vi "dc_motor_drive_pidff.vi"() -> ()   [LabVIEW 2019]
uses:
  <vilib>/myRIO/Common/Instrument Driver Framework/myRIO v1.0/Encoder/typedefs/Encoder Signal Mode.ctl
  <vilib>/myRIO/Instrument Drivers/Onboard IO/Encoder/typedefs/Encoder Reference.ctl
  <vilib>/myRIO/Common/Instrument Driver Framework/Utilities/typedefs/myRIO Generic Hardware Reference.ctl
  <vilib>/myRIO/Common/Instrument Driver Framework/Utilities/typedefs/Hardware Version Enum.ctl
  <vilib>/myRIO/Common/Instrument Driver Framework/Utilities/typedefs/myRIO v1.0 Reference.ctl
  <vilib>/myRIO/Common/Instrument Driver Framework/Utilities/typedefs/Generic FPGA Reference.ctl
  <vilib>/myRIO/Common/Instrument Driver Framework/myRIO v1.0/Encoder/typedefs/Encoder Channels Enum.ctl
  <vilib>/myRIO/Common/Instrument Driver Framework/myRIO v1.0/Encoder/typedefs/Encoder Configuration v1.0.ctl
  <vilib>/userDefined/High Color/nirio_resource_hc.ctl
  <vilib>/Platform/TimedLoop/XDataNode/timing_clust.ctl
  <vilib>/Platform/TimedLoop/XDataNode/nitl_modes.ctl
  <vilib>/Platform/TimedLoop/XDataNode/wakeup.ctl
  <vilib>/myRIO/Instrument Drivers/Onboard IO/PWM/typedefs/PWM Reference.ctl
  <vilib>/myRIO/Common/Instrument Driver Framework/myRIO v1.0/PWM/typedefs/PWM Channels Enum.ctl
  <vilib>/myRIO/Instrument Drivers/Onboard IO/PWM/typedefs/PWM Configuration.ctl
  <vilib>/myRIO/Instrument Drivers/Onboard IO/DIO/typedefs/DIO Reference.ctl
  <vilib>/myRIO/Common/Instrument Driver Framework/myRIO v1.0/DIO/typedefs/DIO Channels List.ctl
  <vilib>/myRIO/Common/Instrument Driver Framework/myRIO v1.0/DIO/typedefs/DIO Channels Enum.ctl
  <vilib>/myRIO/Common/Instrument Driver Framework/Utilities/vis/Is FPGA Ref Available.vi
  <vilib>/myRIO/Common/Instrument Driver Framework/myRIO v1.0/Encoder/vis/myRIO v1.1 Open Encoder.vi
  <vilib>/myRIO/Instrument Drivers/Onboard IO/Encoder/vis/Read.vi
  <vilib>/myRIO/Common/Instrument Driver Framework/myRIO v1.0/PWM/vis/myRIO v1.1 Open PWM.vi
  <vilib>/myRIO/Common/Instrument Driver Framework/myRIO v1.0/DIO/vis/myRIO v1.1 Open DIO.vi
  <vilib>/myRIO/Instrument Drivers/Onboard IO/DIO/vis/Write.vi
  <vilib>/myRIO/Common/Instrument Driver Framework/Utilities/vis/Validate Channels.vi
  <vilib>/myRIO/Common/Instrument Driver Framework/myRIO v1.0/Encoder/vis/myRIO v1.0 Reserve Encoder.vi
  <vilib>/myRIO/Common/Instrument Driver Framework/myRIO v1.0/PWM/vis/myRIO v1.0 Reserve PWM.vi
  <vilib>/myRIO/Common/Instrument Driver Framework/myRIO v1.0/DIO/vis/myRIO v1.0 Reserve DIO.vi
  <vilib>/myRIO/Common/Instrument Driver Framework/myRIO v1.0/Encoder/vis/myRIO v1.0 Build MUX Configuration Encoder.vi
  <vilib>/myRIO/Common/Instrument Driver Framework/myRIO v1.0/Resource Manager/vis/myRIO v1.0 Reserve Channel List.vi
  <vilib>/myRIO/Common/Instrument Driver Framework/myRIO v1.0/PWM/vis/myRIO v1.0 Build MUX Configuration PWM.vi
  <vilib>/myRIO/Common/Instrument Driver Framework/myRIO v1.0/DIO/vis/myRIO v1.0 Build MUX Configuration DIO.vi
  <vilib>/myRIO/Common/Instrument Driver Framework/myRIO v1.0/Resource Manager/vis/myRIO v1.0 Create Configuration List.vi
  <vilib>/myRIO/Common/Instrument Driver Framework/myRIO v1.0/Resource Manager/vis/myRIO v1.0 Reserve Channel.vi
  <vilib>/myRIO/Common/Instrument Driver Framework/myRIO v1.0/Resource Manager/vis/myRIO v1.0 Unreserve Channel.vi
  <vilib>/myRIO/Common/Instrument Driver Framework/myRIO v1.0/Resource Manager/vis/myRIO v1.0 Build Mutex Name.vi
  <vilib>/Utility/VariantDataType/GetNumericInfo.vi
  <vilib>/Utility/error.llb/Error Cluster From Error Code.vi
  <vilib>/myRIO/Common/Instrument Driver Framework/myRIO v1.0/myRIO v1.1 Open.vi
  <vilib>/myRIO/Common/Instrument Driver Framework/Utilities/vis/IO Manager.vi
  <vilib>/myRIO/Common/Instrument Driver Framework/Utilities/vis/Configuration Manager.vi
  <vilib>/myRIO/Common/Instrument Driver Framework/myRIO v1.0/Resource Manager/vis/myRIO v1.0 Configure IO.vi
  <vilib>/myRIO/Common/Instrument Driver Framework/myRIO v1.0/myRIO v1.0 Close.vi
  <vilib>/myRIO/Common/Instrument Driver Framework/myRIO v1.0/Encoder/vis/myRIO v1.0 Configure Encoder.vi
  <vilib>/myRIO/Common/Instrument Driver Framework/myRIO v1.0/Encoder/vis/myRIO v1.0 Read Encoder.vi
  <vilib>/myRIO/Common/Instrument Driver Framework/myRIO v1.0/PWM/vis/myRIO v1.0 Write PWM.vi
  <vilib>/myRIO/Common/Instrument Driver Framework/myRIO v1.0/DIO/vis/myRIO v1.0 Write DIO.vi
  <vilib>/myRIO/Express VI/Onboard IO/Encoder/Encoder Express VI.xnode
  <vilib>/myRIO/Instrument Drivers/Onboard IO/Encoder/vis/myRIO Encoder Open.xnode
  <vilib>/myRIO/Common/Instrument Driver Framework/myRIO v1.0/Encoder/typedefs/Encoder Count Direction Enum.ctl
  <vilib>/Platform/TimedLoop/XDataNode/XDataNode.xnode
  <vilib>/myRIO/Express VI/Onboard IO/PWM/PWM Express VI.xnode
  <vilib>/myRIO/Instrument Drivers/Onboard IO/PWM/vis/myRIO PWM Open.xnode
  <vilib>/myRIO/Express VI/Onboard IO/DO/DO Express VI.xnode
  <vilib>/myRIO/Instrument Drivers/Onboard IO/DIO/vis/myRIO DIO Open.xnode
  <vilib>/myRIO/Instrument Drivers/Onboard IO/PWM/PWM.lvlib
  <vilib>/myRIO/Instrument Drivers/Utilities/Utilities.lvlib
  <vilib>/myRIO/Instrument Drivers/Onboard IO/Encoder/Encoder.lvlib
  <vilib>/Platform/TimedLoop/XDataNode/XDNodeRunTimeDep.lvlib
  <vilib>/myRIO/Instrument Drivers/Onboard IO/DIO/DIO.lvlib
panel:
  out "direction":bool
  out "Angle diff(deg)":dbl(graph)
  out "virtual PWM value":dbl[](graph)
  out "Duty cycle":dbl(graph)
  out "PWM value":i32
  out "Set Point 2":dbl
  out "Set Point":dbl
  out "Setpoint_to_motor":T1
  in  "PWM Max":i32=4096
  in  "gain_ff":T2={"gain_ff 1"={"K_vff"=10000.0, "K_aff"=250.0}, "gain_ff 2"={"K_vff"=10000.0, "K_aff"=250.0}, "gain_ff 3"={"K_vff"=10000.0, "K_aff"=250.0}, "gain_ff 4"={"K_vff"=10000.0, "K_aff"=250.0}, "gain_ff 5"={"K_vff"=10000.0, "K_aff"=250.0}, "gain_ff 6"={"K_vff"=10000.0, "K_aff"=250.0}}
  in  "PIDt":T3={"PID gains 1"={"proportional gain (Kp)"=800.0, "integral time (Ki)"=0.0, "derivative time (Kd)"=1000.0}, "PID gains 2"={"proportional gain (Kp)"=800.0, "integral time (Ki)"=0.0, "derivative time (Kd)"=1000.0}, "PID gains 3"={"proportional gain (Kp)"=800.0, "integral time (Ki)"=0.0, "derivative time (Kd)"=1000.0}, "PID gains 4"={"proportional gain (Kp)"=800.0, "integral time (Ki)"=0.0, "derivative time (Kd)"=1000.0}, "PID gains 5"={"proportional gain (Kp)"=800.0, "integral time (Ki)"=0.0, "derivative time (Kd)"=1000.0}, "PID gains 6"={"proportional gain (Kp)"=800.0, "integral time (Ki)"=0.0, "derivative time (Kd)"=1000.0}}
  in  "PWM value":T4 {"PWM value 6" scale=0.0..4096.0; "PWM value 5" scale=0.0..4096.0; "PWM value 4" scale=0.0..4096.0; "PWM value 3" scale=0.0..4096.0; "PWM value 2" scale=0.0..4096.0; "PWM value 1" scale=0.0..4096.0}
  out "time":dbl
  out "Angle_velocity(deg/s)":cluster{"set point":dbl, dbl}(graph)
  out "Angle_velocity(deg) Graph":dbl[][](graph)
  out "Angle(deg) Graph":dbl[][](graph)
  out "Angle(deg)":cluster{dbl, dbl}(graph)
  in  "DC motor stop":bool
  in  "Frequency [Hz]":dbl=1000.0
  out "encoder_position":dbl
  out "Counter Value":i32
  in  "Encoder_Count":dbl=54991.0
  in  "t_shift":dbl=0.000125
  in  "T_ratio":dbl=10.0
  in  "buffer ratio":dbl=0.3
  in  "first or second tripod":bool
  in  "data of 5th order formula\nts,tair,a1-a6":dbl[](array[numeric])
  in  "Loop Period":i64=5
  out "duty cycle[%]":dbl
  out "pulse width[ms]":dbl
  in  "frequency":dbl=100.0
  out "offset":dbl
  in  "null offset":bool
  in  "position":dbl(slide) scale=-30.0..8.0
  in  "PWM channel":tag="A/PWM1"
  in  "RC motor stop":bool
  # "DC Motor"
  # "RC Servo Motor"
  # "v = 1; a = 15"
  # "v = 1.25; a = 15"
  # "v = 1.5; a = 15"
  # "0.184067181524967\n0.263820978418769\n256152.551336786\n-30272.30000274\n-9876.03760433421\n-1096.38594197941\n885.91817900106\n-44.6781799901984"
  # "0.215241998794118\n0.254514142390288\n4771.41078363533\n62185.8763006578\n-22508.5336527453\n390.805502041188\n686.695311017595\n-40.4128145310291"
  # "0.163616269216122\n0.27489641502463\n771965.39318528\n-201617.027694185\n8828.08396944145\n-2683.04589908678\n1085.57303422127\n-48.5860395324432"
  # "v = 1.75; a = 15"
  # "v = 2; a = 15"
  # "v = 2.25; a = 15"
  # "0.148651048423414\n0.288542414074344\n1776973.44893281\n-511591.467559457\n38775.9830765103\n-4576.94506688942\n1289.39828252671\n-52.3115561007577"
  # "0.136976185169818\n0.304016701267508\n3461279.85083822\n-993110.73746345\n80544.6579529191\n-6699.48295844177\n1494.82265451498\n-55.8934424469099"
  # "0.134381902205816\n0.369022171779704\n3272804.8365432\n-899365.569589567\n71225.2463409934\n-7039.10791102172\n1512.66147498591\n-59.3408899720725"
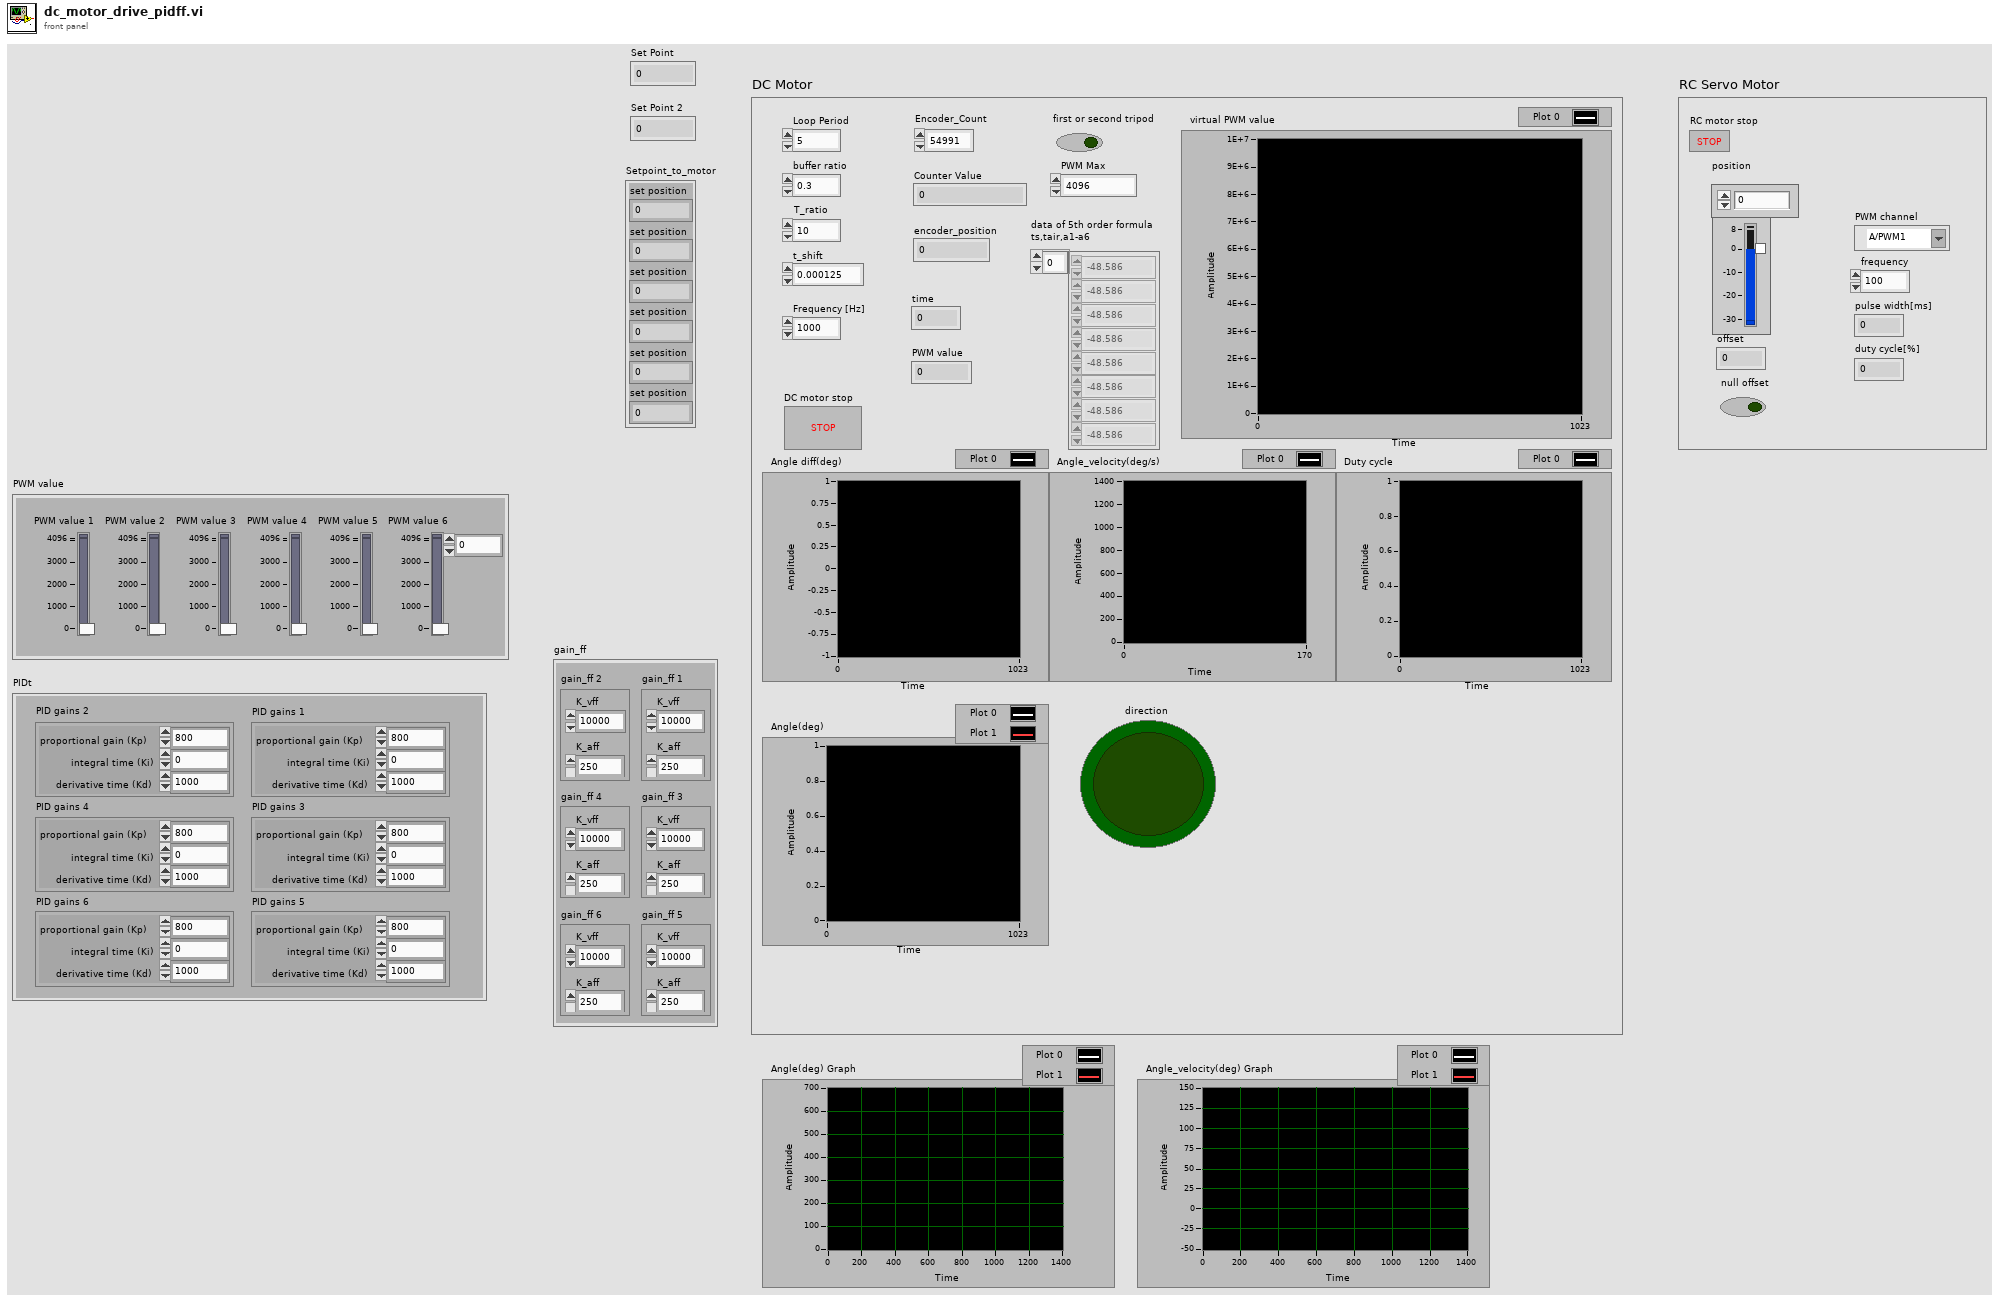
[diagram p1: front panel]
types:
  T1 = cluster{"set position":dbl, "set position":dbl, "set position":dbl, "set position":dbl, "set position":dbl, "set position":dbl}
  T2 = cluster{"gain_ff 1":cluster{"K_vff":dbl, "K_aff":dbl}, "gain_ff 2":cluster{"K_vff":dbl, "K_aff":dbl}, "gain_ff 3":cluster{"K_vff":dbl, "K_aff":dbl}, "gain_ff 4":cluster{"K_vff":dbl, "K_aff":dbl}, "gain_ff 5":cluster{"K_vff":dbl, "K_aff":dbl}, "gain_ff 6":cluster{"K_vff":dbl, "K_aff":dbl}}
  T3 = cluster{"PID gains 1":cluster{"proportional gain (Kp)":dbl, "integral time (Ki)":dbl, "derivative time (Kd)":dbl}, "PID gains 2":cluster{"proportional gain (Kp)":dbl, "integral time (Ki)":dbl, "derivative time (Kd)":dbl}, "PID gains 3":cluster{"proportional gain (Kp)":dbl, "integral time (Ki)":dbl, "derivative time (Kd)":dbl}, "PID gains 4":cluster{"proportional gain (Kp)":dbl, "integral time (Ki)":dbl, "derivative time (Kd)":dbl}, "PID gains 5":cluster{"proportional gain (Kp)":dbl, "integral time (Ki)":dbl, "derivative time (Kd)":dbl}, "PID gains 6":cluster{"proportional gain (Kp)":dbl, "integral time (Ki)":dbl, "derivative time (Kd)":dbl}}
  T4 = cluster{"PWM value 1":i32, "PWM value 2":i32, "PWM value 3":i32, "PWM value 4":i32, "PWM value 5":i32, "PWM value 6":i32}
  T5 = typedef "Encoder.lvlib/Encoder Reference.ctl" = cluster{"myRIO Reference":T6, "Encoder Channels Enum":T10}
  T6 = typedef "myRIO Generic Hardware Reference.ctl" = cluster{"myRIO Model":T7, "myRIO Hardware Reference":T8}
  T7 = typedef "Hardware Version Enum.ctl" = enum16{"Unknown", "myRIO-1900", "myRIO-1950", "roboRIO", "NI ELVIS RIO CM", "ELVIS III"}
  T8 = typedef "myRIO v1.0 Reference.ctl" = cluster{"Generic FPGA Reference":T9, "Allow multiple opens":bool}
  T9 = typedef "Generic FPGA Reference.ctl" = refnum<k20>
  T10 = typedef "Encoder Channels Enum.ctl" = enum16{"Not Connected", "C/ENC0", "C/ENC1", "A/ENC", "A/ENC0", "A/ENC1", "A/ENC2", "A/ENC3", "A/ENC4", "A/ENC5", "A/ENC6", "A/ENC7", "A/ENC8", "A/ENC9", "B/ENC", "B/ENC0", "B/ENC1", "B/ENC2", "B/ENC3", "B/ENC4", "B/ENC5", "B/ENC6", "B/ENC7", "B/ENC8", "B/ENC9", "DIO/ENC0", "DIO/ENC1", "DIO/ENC2", "DIO/ENC3", "DIO/ENC4"}
  T11 = typedef "Encoder Signal Mode.ctl" = enum16{"Quadrature phase signal", "Step and direction signal"}
  T12 = typedef "nirio_resource_hc.ctl" = tag
  T13 = cluster{"setPWM":bool, "setPWM":bool, "setPWM":bool, "setPWM":bool, "setPWM":bool, "setPWM":bool}
  T14 = typedef "DIO.lvlib/DIO Reference.ctl" = cluster{"myRIO Reference":T6, "DIO Channels List":T15}
  T15 = typedef "DIO Channels List.ctl" = T16[]
  T16 = typedef "DIO Channels Enum.ctl" = enum16{"Not Connected", "C/DIO0", "C/DIO1", "C/DIO2", "C/DIO3", "C/DIO4", "C/DIO5", "C/DIO6", "C/DIO7", "A/DIO0", "A/DIO1", "A/DIO2", "A/DIO3", "A/DIO4", "A/DIO5", "A/DIO6", "A/DIO7", "A/DIO8", "A/DIO9", "A/DIO10", "A/DIO11", "A/DIO12", "A/DIO13", "A/DIO14", "A/DIO15", "A/DIO16", "A/DIO17", "A/DIO18", "A/DIO19", "B/DIO0", "B/DIO1", "B/DIO2", "B/DIO3", "B/DIO4", "B/DIO5", "B/DIO6", "B/DIO7", "B/DIO8", "B/DIO9", "B/DIO10", "B/DIO11", "B/DIO12", "B/DIO13", "B/DIO14", "B/DIO15", "B/DIO16", "B/DIO17", "B/DIO18", "B/DIO19", "LED0", "LED1", "LED2", "LED3", "Button0", "DIO/DIO0", "DIO/DIO1", "DIO/DIO2", "DIO/DIO3", "DIO/DIO4", "DIO/DIO5", "DIO/DIO6", "DIO/DIO7", "DIO/DIO8", "DIO/DIO9", "SPI/CS0", "SPI/CS1", "SPI/CS2", "SPI/CS3", "LED RADIO (Green)", "LED RADIO (Red)", "LED COMM (Green)", "LED COMM (Red)", "LED MODE (Green)", "LED MODE (Red)"}
  T17 = typedef "PWM.lvlib/PWM Reference.ctl" = cluster{"myRIO Reference":T6, "PWM Channels Enum":T18, "PWM Configuration":T19}
  T18 = typedef "PWM Channels Enum.ctl" = enum16{"Not Connected", "C/PWM0", "C/PWM1", "A/PWM0", "A/PWM1", "A/PWM2", "A/PWM3", "A/PWM4", "A/PWM5", "A/PWM6", "A/PWM7", "A/PWM8", "A/PWM9", "A/PWM10", "A/PWM11", "A/PWM12", "A/PWM13", "A/PWM14", "A/PWM15", "A/PWM16", "A/PWM17", "A/PWM18", "A/PWM19", "B/PWM0", "B/PWM1", "B/PWM2", "B/PWM3", "B/PWM4", "B/PWM5", "B/PWM6", "B/PWM7", "B/PWM8", "B/PWM9", "B/PWM10", "B/PWM11", "B/PWM12", "B/PWM13", "B/PWM14", "B/PWM15", "B/PWM16", "B/PWM17", "B/PWM18", "B/PWM19", "PWM/PWM0", "PWM/PWM1", "PWM/PWM2", "PWM/PWM3", "PWM/PWM4", "PWM/PWM5", "PWM/PWM6", "PWM/PWM7", "PWM/PWM8", "PWM/PWM9"}
  T19 = typedef "PWM.lvlib/PWM Configuration.ctl" = cluster{"Frequency":dbl, "Duty Cycle":dbl}
  T20 = typedef "XDNodeRunTimeDep.lvlib/timing_clust.ctl" = cluster{"Expected End [f-1]":u64, "Actual End [f-1]":u64, "Finished Late? [f-1]":bool, "Expected End [i-1]":u64, "Actual End [i-1]":u64, "Finished Late? [i-1]":bool, "Expected Start [i]":u64, "Actual Start [i]":u64, "Expected Start [f]":u64, "Actual Start [f]":u64, "Source Name":string, "Structure Name":string, "Period":i64, "Deadline":i64, "Offset":i64, "Start":i64, "Priority":i32, "Timeout":i32, "Mode":T21, "Wakeup Reason":T22, "Error":errorcluster, "Source Type":string, "Secondary Source Type":string, "Global End Time":u64, "Global Start Time":u64, "Frame Duration":u64, "Iteration Duration":u64, "Assigned CPU":i32, "I/O Scan Engine Mode":u32}
  T21 = typedef "XDNodeRunTimeDep.lvlib/nitl_modes.ctl" = enum32{"No Change", "Process missed periods, maintain original phase", "Discard missed periods, maintain original phase", "Process missed periods, ignore original phase", "Discard missed periods, ignore original phase"}
  T22 = typedef "XDNodeRunTimeDep.lvlib/wakeup.ctl" = enum32{"Normal", "Aborted", "Asynchronous wakeup", "Timing source error", "Timed loop error", "Timeout"}
  T23 = cluster{"A_ff Rfr":dbl, "A_ff Lfr 2":dbl, "A_ff Rm 2":dbl, "A_ff Lm":dbl, "A_ff Rfr":dbl, "A_ff Lfr 2":dbl}
  T24 = cluster{"Set Point (V) Rfr":dbl, "Set Point (V) Lfr 2":dbl, "Set Point (V) Rm 2":dbl, "Set Point (V) Lm":dbl, "Set Point (V) Rfr":dbl, "Set Point (V) Lfr 2":dbl}
  T25 = cluster{"[0]":dbl, "[1]":dbl, "[2]":dbl, "[3]":dbl, "[4]":dbl, "[5]":dbl}
  T26 = cluster{"set position":i32, "set position":i32, "set position":i32, "set position":i32, "set position":i32, "set position":i32}
  T27 = cluster{"proportional gain (Kp)":dbl, "integral time (Ki)":dbl, "derivative time (Kd)":dbl}[]
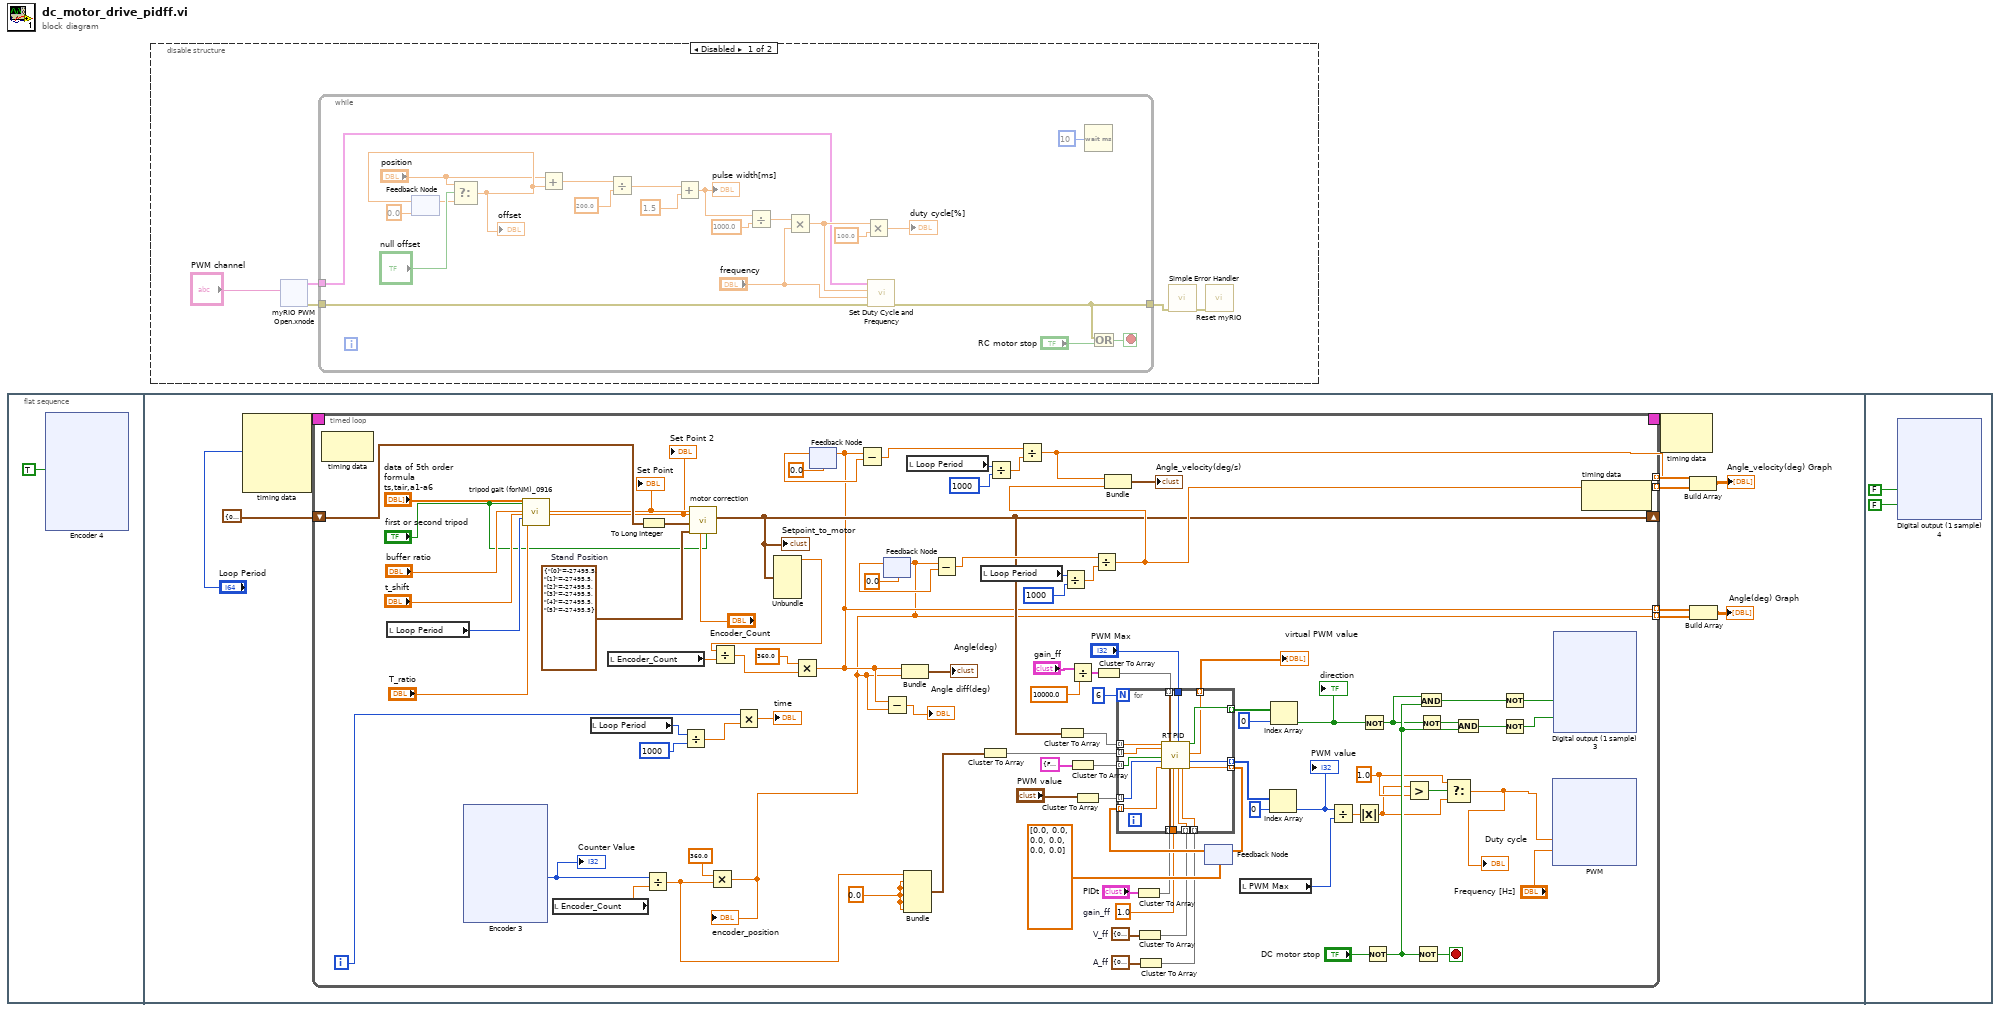
[diagram p0: block diagram]
diagram:
  n1 = flat-sequence {
    frame #0 {
      n2 = xnode "Encoder 4"("Reset Counter"=TRUE) -> ()  [unwired: 1 in, 4 out]
    }
    frame #1 {
      n3 = node-c288("Loop Period") -> (w57:T20)  [unwired: 3 in]
      n4 = timed-loop {
        timing: w57 -> [_]
        timing-out: [_] -> w56
        shift-right: [w76] -> _
        shift-left: T1 {"set position"=0.0, "set position"=0.0, "set position"=0.0, "set position"=0.0, "set position"=0.0, "set position"=0.0} ("Setpoint_to_motor") -> [w139]
        tunnel: [w59] -> w52 mode=indexing
        tunnel: [w60] -> w53 mode=indexing
        tunnel: [w106] -> w50 mode=indexing
        tunnel: [w105] -> w49 mode=indexing
        i -> [w99]
        stop <- w125 stop-if-true
        w69 = 0.0
        w83 = T23 {"A_ff Rfr"=0.0, "A_ff Lfr 2"=0.0, "A_ff Rm 2"=0.0, "A_ff Lm"=0.0, "A_ff Rfr"=0.0, "A_ff Lfr 2"=0.0}  # A_ff
        w85 = T24 {"Set Point (V) Rfr"=0.0, "Set Point (V) Lfr 2"=0.0, "Set Point (V) Rm 2"=0.0, "Set Point (V) Lm"=0.0, "Set Point (V) Rfr"=0.0, "Set Point (V) Lfr 2"=0.0}  # V_ff
        w86 = 1.0  # gain_ff
        w132 = 1.0 ("y")
        w138 = T25 {"[0]"=-27495.5, "[1]"=-27495.5, "[2]"=-27495.5, "[3]"=-27495.5, "[4]"=-27495.5, "[5]"=-27495.5}  # Stand Position
        n5 = node-c288() -> ()  [unwired: 1 in, 1 out]
        n6 = local read "Loop Period"() -> (w145:i64)
        n7 = xnode "Encoder 3"() -> ("Counter Value"=w141:i32)  [unwired: 2 in, 3 out]
        "Counter Value" <- w141
        n8 = call "tripod gait (forNM)_0916.vi"("data of 5th order formula\nts,tair,a1-a6"="data of 5th order formula\nts,tair,a1-a6", "first or second"="first or second tripod", "buffer ratio"="buffer ratio", "t_shift"="t_shift", "sample time"=w145, "T_ratio"="T_ratio") -> ("Set Point"=w103:dbl, "Set Point 2"=w102:dbl)  [unwired: 4 in, 16 out]
        "Set Point" <- w103
        "Set Point 2" <- w102
        n9 = local read "Encoder_Count"() -> (w142:dbl)
        n10 = local read "Loop Period"() -> (w112:i64)
        n11 = local read "Encoder_Count"() -> (w110:dbl)
        n12 = To Long Integer(number=w139) -> (32bit integer=w140:T26)
        n13 = Divide(x=w141, y=w142) -> (x/y=w68:dbl)
        n14 = Divide(x=w112, y=i64 1000) -> (x/y=w100:dbl)
        n15 = call "motor correction.vi"("first or second"="first or second tripod", "Encoder_Count"="Encoder_Count", "Stand Position"=w138, "encoder position"=w140, "set position 2"=w102, "set position"=w103) -> ("Setpoint_to_motor"=w76:T1)  [unwired: 4 in, 1 out]
        "Setpoint_to_motor" <- w76
        n16 = Multiply(x=360.0, y=w68) -> (x*y=w59:dbl)
        "encoder_position" <- w59
        n17 = Multiply(x=w99, y=w100) -> (x*y=→"time":dbl)
        n18 = Unbundle(w76) -> ("set position"=w97:dbl)  [unwired: 5 out]
        n19 = Divide(x=w97, y=w110) -> (x/y=w108:dbl)
        n20 = Multiply(x=360.0, y=w108) -> (x*y=w60:dbl)
        n21 = feedback #1(0.0) -> (w118:dbl)
        n22 = feedback-in #1(w60) -> ()
        n23 = Subtract(x=w60, y=w118) -> (x-y=w114:dbl)
        n24 = feedback #2(0.0) -> (w123:dbl)
        n25 = feedback-in #2(w59) -> ()
        n26 = Subtract(x=w60, y=w59) -> (x-y=→"Angle diff(deg)":dbl)
        n27 = Bundle(w60, w59) -> (→"Angle(deg)":cluster{dbl, dbl})  [unwired: 1 in]
        n28 = Bundle(w68, w69, w69, w69, w69, w69) -> (w71:cluster{dbl, dbl, dbl, dbl, dbl, dbl})  [unwired: 1 in]
        n29 = local read "Loop Period"() -> (w117:i64)
        n30 = Subtract(x=w59, y=w123) -> (x-y=w119:dbl)
        n31 = local read "Loop Period"() -> (w122:i64)
        n32 = Cluster To Array(cluster=w71) -> (array=w70:dbl[])
        n33 = Divide(x=w117, y=i64 1000) -> (x/y=w115:dbl)
        n34 = Divide(x=w114, y=w115) -> (x/y=w105:dbl)
        n35 = Cluster To Array(cluster=w76) -> (array=w75:dbl[])
        n36 = Divide(x=w122, y=i64 1000) -> (x/y=w120:dbl)
        n37 = Divide(x="gain_ff", y=10000.0) -> (x/y=w79:T2)
        n38 = Cluster To Array(cluster=T13 {"setPWM"=FALSE, "setPWM"=FALSE, "setPWM"=FALSE, "setPWM"=FALSE, "setPWM"=FALSE, "setPWM"=FALSE}) -> (array=w94:bool[])
        n39 = Cluster To Array(cluster="PWM value") -> (array=w92:i32[])
        n40 = Divide(x=w119, y=w120) -> (x/y=w106:dbl)
        n41 = Cluster To Array(cluster=w79) -> (array=w78:cluster{"K_vff":dbl, "K_aff":dbl}[])
        n42 = Bundle(w105, w106) -> (→"Angle_velocity(deg/s)":cluster{dbl, dbl})  [unwired: 1 in]
        n43 = Cluster To Array(cluster="PIDt") -> (array=w87:T27)
        n44 = Cluster To Array(cluster=w85) -> (array=w84:dbl[])
        n45 = Cluster To Array(cluster=w83) -> (array=w82:dbl[])
        n46 = feedback #3(dbl[] [0.0, 0.0, 0.0, 0.0, 0.0, 0.0]) -> (w91:dbl[])
        n47 = for {
          N: 6 -> [_]
          tunnel: w94 -> [w164] mode=indexing
          tunnel: w92 -> [w163] mode=indexing
          tunnel: w91 -> [w162] mode=indexing
          tunnel: [w161] -> w90 mode=indexing
          tunnel: w87 -> [w160] mode=indexing
          tunnel: w86 -> [w159]
          tunnel: w84 -> [w158] mode=indexing
          tunnel: w82 -> [w157] mode=indexing
          tunnel: w78 -> [w156] mode=indexing
          tunnel: "PWM Max" -> [w155]
          tunnel: w75 -> [w154] mode=indexing
          tunnel: [w153] -> w74 mode=indexing
          tunnel: w70 -> [w152] mode=indexing
          tunnel: [w151] -> w66 mode=indexing
          tunnel: [w150] -> w61 mode=indexing
          n48 = call "RT PID.vi"("setpoint"=w154, "Encoder"=w152, "set PWM"=w164, "PWM value"=w163, "last error"=w162, 6:"gain_ff"=w156, "PID"=w160, 9:"gain_ff"=w159, "PWM Max"=w155, "V_ff"=w158, "A_ff"=w157) -> ("direction"=w153:bool, "PWM value"=w150:dbl, "PWM"=w151:i32, "error"=w161:dbl)  [unwired: 2 in, 3 out]
        }
        "virtual PWM value" <- w61
        n49 = feedback-in #3(w90) -> ()
        n50 = local read "PWM Max"() -> (w65:i32)
        n51 = Index Array(array=w66, index=0) -> (element=w62:i32)
        "PWM value" <- w62
        n52 = Index Array(array=w74, index=0) -> (element=w72:bool)
        "direction" <- w72
        n53 = Divide(x=w62, y=w65) -> (x/y=w64:dbl)
        n54 = Absolute Value(x=w64) -> (abs(x)=w131:dbl)
        n55 = Not(x=w72) -> (.not. x?=w130:bool)
        n56 = Not(x="DC motor stop") -> (.not. x?=w134:bool)
        n57 = Greater?(x=w131, y=w132) -> (0:w133:bool)
        n58 = Not(x=w134) -> (.not. x?=w125:bool)
        n59 = And(x=w130, y=w134) -> (x .and. y?=w127:bool)
        n60 = Not(x=w130) -> (.not. x?=w136:bool)
        n61 = Select(t=w132, s=w133, f=w131) -> (s? t:f=w63:dbl)
        "Duty cycle" <- w63
        n62 = And(x=w136, y=w134) -> (x .and. y?=w129:bool)
        n63 = Not(x=w127) -> (.not. x?=w126:bool)
        n64 = Not(x=w129) -> (.not. x?=w128:bool)
        n65 = xnode "PWM"("Duty Cycle"=w63, "Frequency [Hz]"="Frequency [Hz]") -> ()  [unwired: 1 in, 1 out]
        n66 = xnode "Digital output (1 sample) 3"("A/DIO0 (Pin 11)"=w126, "A/DIO1 (Pin 13)"=w128) -> ()  [unwired: 1 in, 1 out]
        n67 = node-c288() -> ()  [unwired: 1 in, 1 out]
      }
      n68 = node-c288(w56) -> ()  [unwired: 1 out]
      n69 = Build Array(w49, w50) -> (→"Angle_velocity(deg) Graph":dbl[][])
      n70 = Build Array(w53, w52) -> (→"Angle(deg) Graph":dbl[][])
    }
    frame #2 {
      n71 = xnode "Digital output (1 sample) 4"("A/DIO0 (Pin 11)"=FALSE, "A/DIO1 (Pin 13)"=FALSE) -> ()  [unwired: 1 in, 1 out]
    }
  }
  n72 = disable-structure shown="Disabled" {
    frame Disabled {
      n73 = xnode "myRIO PWM Open.xnode"("Channel Name"="PWM channel") -> ("error out"=w328:errorcluster, "PWM Ref Out"=w329:T17)  [unwired: 2 in]
      n74 = while {
        tunnel: w329 -> [w353]
        tunnel: w328 -> [w352]
        tunnel: [w351] -> w327
        stop <- w349 stop-if-true
        n75 = feedback #4(0.0 ("Numeric")) -> (w366:dbl)
        n76 = Select(t="position", s="null offset", f=w366) -> (s? t:f=w365:dbl)
        "offset" <- w365
        n77 = feedback-in #4(w365) -> ()
        n78 = Add(x="position", y=w365) -> (x+y=w364:dbl)
        n79 = Divide(x=w364, y=200.0) -> (x/y=w362:dbl)
        n80 = Add(x=w362, y=1.5) -> (x+y=w360:dbl)
        "pulse width[ms]" <- w360
        n81 = Divide(x=w360, y=1000.0) -> (x/y=w358:dbl)
        n82 = Multiply(x=w358, y="frequency") -> (x*y=w356:dbl)
        n83 = Multiply(x=w356, y=100.0) -> (x*y=→"duty cycle[%]":dbl)
        n84 = call <vilib>:"Set Duty Cycle and Frequency.vi"("error in (no error)"=w352, "Frequency [Hz]"="frequency", "Duty Cycle"=w356, "PWM Ref In"=w353) -> ("error out"=w351:errorcluster)  [unwired: 5 in, 1 out]
        n85 = Wait (ms)(milliseconds to wait=u32 10) -> ()  [unwired: 1 out]
        n86 = Or(x=w351, y="RC motor stop") -> (x .or. y?=w349:bool)
      }
      n87 = call <vilib>:"Simple Error Handler.vi"("error in (no error)"=w327) -> ("error out"=w326:errorcluster)  [unwired: 4 in, 4 out]
      n88 = call <vilib>:"Reset myRIO.vi"("error in (no error)"=w326) -> ()  [unwired: 10 in, 1 out]
    }
    frame Enabled {
    }
  }
